vi "set_Ic_sim_parameter.vi"(8 "error in (no error)":errorcluster, 10 "Parameters":T1 {"temperature K" step=0.01}, 11 "path in":path) -> (0 "error out":errorcluster, 3 "path out":path)   [LabVIEW 2023]
uses:
  paramaters2.ctl
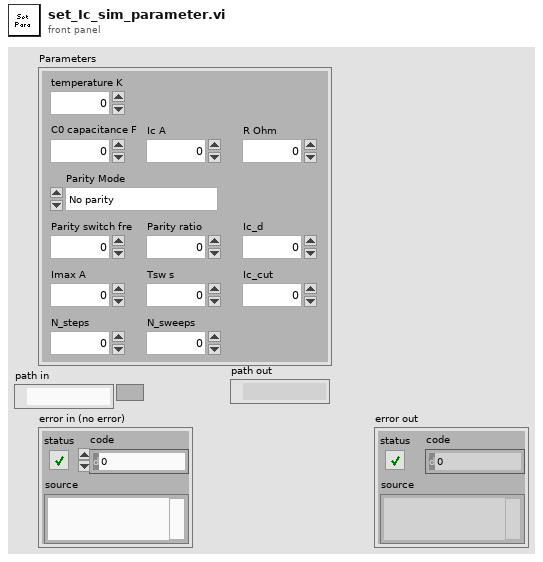
[diagram p1: front panel]
types:
  T1 = typedef "paramaters2.ctl" = cluster{"temperature K":dbl, "C0 capacitance F":dbl, "Ic A":dbl, "R Ohm":dbl, "Parity Mode":enum16{"No parity", "Parity with random lifetime", "For Ic-Ic_d/2", "For Ic+Ic_d/2", "Parity with constant lifetime"}, "Parity switch fre":dbl, "Parity ratio":dbl, "Imax A":dbl, "Tsw s":dbl, "N_steps":i32, "Ic_d":dbl, "N_sweeps":i32, "Ic_cut":dbl}
  T2 = enum16{"No parity", "Parity with random lifetime", "For Ic-Ic_d/2", "For Ic+Ic_d/2", "Parity with constant lifetime"}
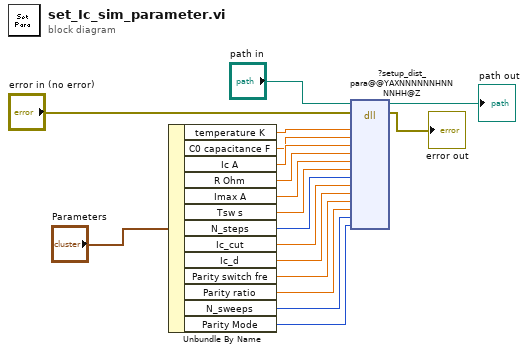
[diagram p0: block diagram]
diagram:
  n1 = Unbundle By Name("Parameters") -> ("temperature K"=w5:dbl, "C0 capacitance F"=w6:dbl, "Ic A"=w7:dbl, "R Ohm"=w8:dbl, "Imax A"=w9:dbl, "Tsw s"=w10:dbl, "N_steps"=w11:i32, "Ic_cut"=w12:dbl, "Ic_d"=w13:dbl, "Parity switch fre"=w14:dbl, "Parity ratio"=w15:dbl, "N_sweeps"=w16:i32, "Parity Mode"=w17:T2)
  n2 = dll-call lib="C:/Users/gyue/Box/Guang Yue uiuc research box folder/computation/Labview simulation GUI/ygDLL.dll" fn="?setup_dist_para@@YAXNNNNNNHNNNNHH@Z"(path in="path in", error in="error in (no error)", "temp"=w5, "c"=w6, "ic"=w7, "r"=w8, "im"=w9, "tsw"=w10, "nstep"=w11, "lcut"=w12, "ic_d"=w13, "fparity"=w14, "icr"=w15, "sweeps"=w16, "mode"=w17) -> (path out=→"path out":path, error out=→"error out":errorcluster)  [unwired: 15 in]
